vi "Configure Gate View (Frequency Sweep).vi"(0 "VISA resource name":refnum<visa-resource-name>, 1 "Gate View Detection Mode (0:Normal)":i32(ring) items=["Normal", "Positive", "Negative", "Sample", "RMS"], 2 "Enable Gate View Detection (T:Enable)":bool=TRUE, 5 "Enable Center Frequency Mode (T:Enable)":bool=TRUE, 7 "Center Frequency (100000000Hz)":dbl=100000000.0 min=-100000000.0 max=43100000000.0, 9 "Sweep Time (1E-6s)":dbl=1e-06 min=1e-06 max=1000.0 format="%#_12g", 11 "error in (no error)":errorcluster, 12 "Sweep Points (3:10001)":i32(ring)=3 items=["1001", "2001", "5001", "10001"]) -> (4 "VISA resource name out":refnum<visa-resource-name>, 15 "error out":errorcluster)   [LabVIEW 2020, in "Anritsu Signal Analyzer Series.lvlib"]
doc: "Configures the gate view(Frequency and Sweep) settings of the spectrum analyzer."
uses:
  Anritsu Signal Analyzer Series.lvlib
panel:
  # "Hz"
  # "s"
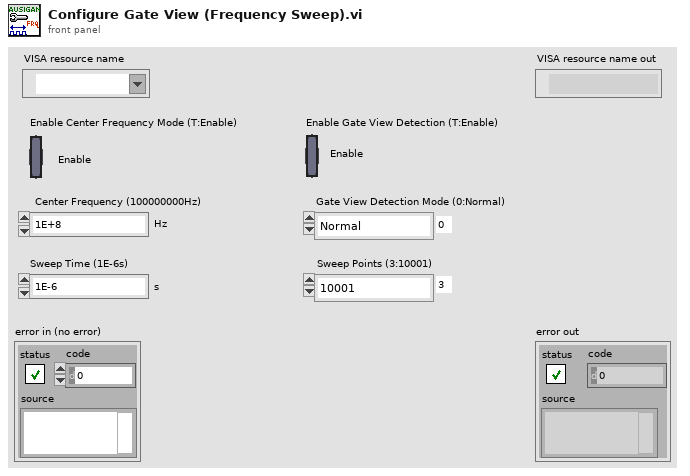
[diagram p1: front panel]
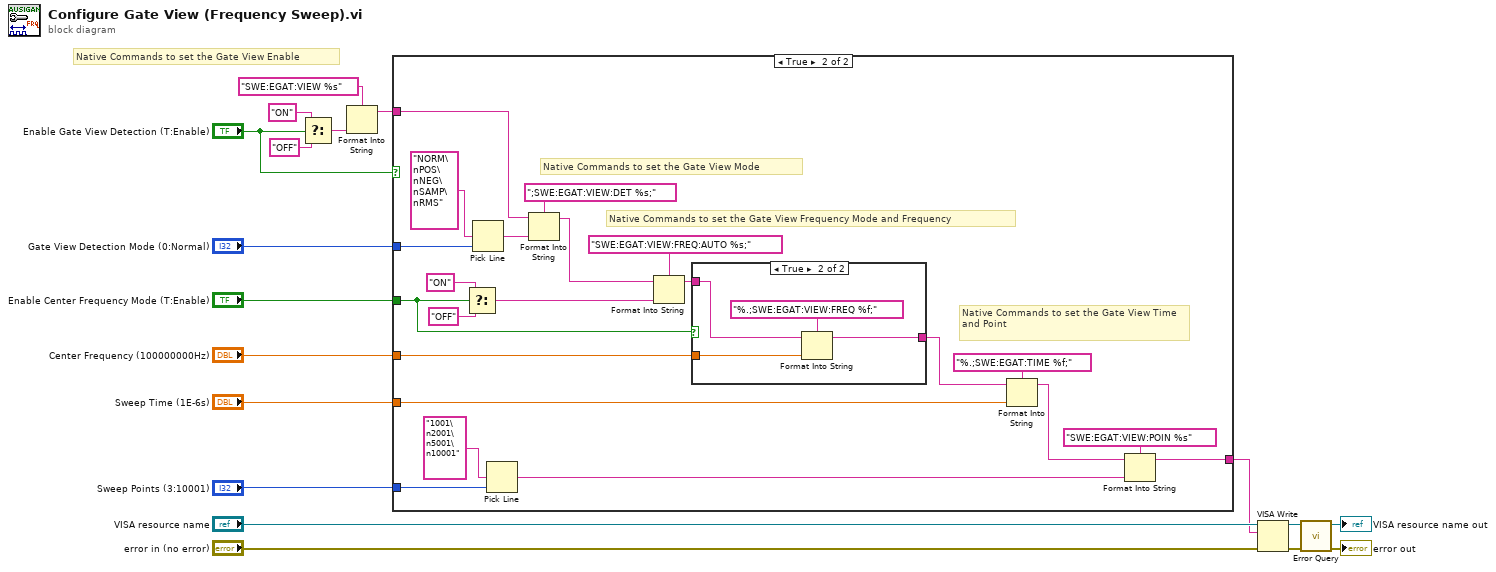
[diagram p0: block diagram]
diagram:
  # "Native Commands to set the Gate View Enable"
  n1 = Select(t="ON" ("string"), s="Enable Gate View Detection (T:Enable)", f="OFF" ("string")) -> (s? t:f=w2:string)
  n2 = Format Into String(format string="SWE:EGAT:VIEW %s" ("_CommandSet"), w2) -> (resulting string=w6:string)  [unwired: 2 in, 1 out]
  n3 = case shown="True" "Enable Gate View Detection (T:Enable)" {
    tunnel: "Gate View Detection Mode (0:Normal)" -> [_ w25]
    tunnel: w6 -> [w19 w41]
    tunnel: "Enable Center Frequency Mode (T:Enable)" -> [_ w23]
    tunnel: "Center Frequency (100000000Hz)" -> [_ w36]
    tunnel: "Sweep Time (1E-6s)" -> [_ w33]
    tunnel: "Sweep Points (3:10001)" -> [_ w20]
    tunnel: [w19 w30] -> w5
    frame False {
    }
    frame True {
      # "Native Commands to set the Gate View Time and Point"
      # "Native Commands to set the Gate View Frequency Mode and Frequency"
      # "Native Commands to set the Gate View Mode"
      n4 = Select(t="ON" ("string"), s=w23, f="OFF" ("string")) -> (s? t:f=w27:string)
      n5 = Pick Line(multi-line string="NORM\nPOS\nNEG\nSAMP\nRMS" ("string"), line index=w25) -> (output string=w24:string)  [unwired: 1 in]
      n6 = Pick Line(multi-line string="1001\n2001\n5001\n10001" ("_Case0"), line index=w20) -> (output string=w21:string)  [unwired: 1 in]
      n7 = Format Into String(format string=";SWE:EGAT:VIEW:DET %s;" ("_CommandSet"), initial string=w41, w24) -> (resulting string=w39:string)  [unwired: 1 in, 1 out]
      n8 = Format Into String(format string="SWE:EGAT:VIEW:FREQ:AUTO %s;" ("_CommandSet"), initial string=w39, w27) -> (resulting string=w37:string)  [unwired: 1 in, 1 out]
      n9 = case shown="True" w23 {
        tunnel: w37 -> [w42 w46]
        tunnel: w36 -> [_ w44]
        tunnel: [w42 w43] -> w35
        frame False {
        }
        frame True {
          n10 = Format Into String(format string="%.;SWE:EGAT:VIEW:FREQ %f;" ("_CommandSet"), initial string=w46, w44) -> (resulting string=w43:string)  [unwired: 1 in, 1 out]
        }
      }
      n11 = Format Into String(format string="%.;SWE:EGAT:TIME %f;" ("_CommandSet"), initial string=w35, w33) -> (resulting string=w32:string)  [unwired: 1 in, 1 out]
      n12 = Format Into String(format string="SWE:EGAT:VIEW:POIN %s", initial string=w32, w21) -> (resulting string=w30:string)  [unwired: 1 in, 1 out]
    }
  }
  n13 = VISA Write(VISA resource name="VISA resource name", write buffer=w5, error in (no error)="error in (no error)") -> (VISA resource name out=w8:refnum<visa-resource-name>, error out=w7:errorcluster)  [unwired: 1 out]
  n14 = call "Error Query.vi"("error in (no error)"=w7, "VISA resource name"=w8) -> ("error out"=→"error out":errorcluster, "VISA resource name out"=→"VISA resource name out":refnum<visa-resource-name>)  [unwired: 6 in, 2 out]
